vi "FVT (New Counter).vi"() -> ()   [LabVIEW 2024]
uses:
  Agilent 532XX Series/Public/Configure/Measurement/Configure Measurement (Frequency).vi
  <vilib>/Utility/file.llb/Write Delimited Spreadsheet (string).vi
  Agilent 532XX Series/Agilent 532XX Series.lvlib
panel:
  out "FrequencyCounter":refnum<visa-resource-name>
  in  "CompRun":bool
  out "Channel(s) (out)":u16(ring) items=["1+2", "1", "2", "3"]
  in  "Single Func Test":bool=TRUE
  in  "Position":i32 min=0 max=64 step=32
  in  "Number of Cycles":i32
  in  "Warmup Data":string[](array[string])
  out "Nominal Frequency":string="XXXXX-XXX"
  in  "Warmup":bool=TRUE
  out "Soak Time":u16(ring) items=["10", "5", "15", "30", "60", "90", "120"]
  out "Starting Time":string
  in  "Slew Time":dbl=2.0 format="%#_13g"
  out "Time Left (Estimate)":string
  out "Time":dbl
  out "PDF Path":string
  out "Time Start":timestamp
  in  "Halt Run":bool=TRUE
  out "Gatetime":string
  out "Delay Time":dbl
  out "Work Order":string
  out "Unit_Number":string
  out "System":string
  out "Path":string
  out "Frequency Address":i16=8
  out "HP Switcher Address":i32=3
  out "Oven Address":i32
  out "Temperature Array":dbl[](array[numeric])
  out "Temp Type":i32 min=1 max=15 step=1
  in  "Serial Numbers":string[](array[string])
  out "All Data":string[][][](array[string])
  in  "System Status":string
  out "Chamber":cluster{"GPIB #":u8, "Address":u8}={"GPIB #"=0, "Address"=28}
  in  "Exit":bool=TRUE
  out "Functional Test Data":string
  in  "Number of Units":i32 min=0 max=64 step=32
  in  "Functional Test":bool=TRUE
  in  "Start run":bool=TRUE
  # "FVT Test Chamber 3"
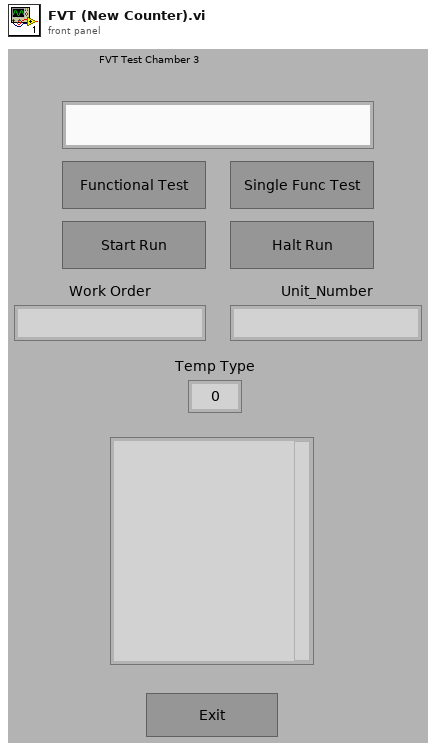
[diagram p1: front panel]
types:
  T1 = cluster{"GPIB Bus":i32, "HP Switcher Address":i32}
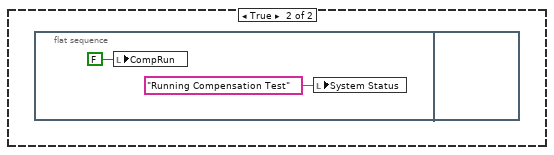
[diagram p2: hidden frame]
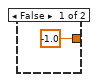
[diagram p4: hidden frame]
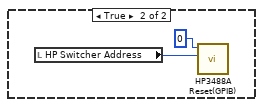
[diagram p5: hidden frame]
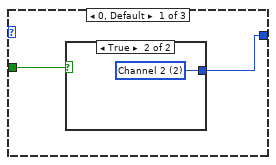
[diagram p6: hidden frame]
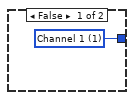
[diagram p7: hidden frame]
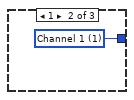
[diagram p8: hidden frame]
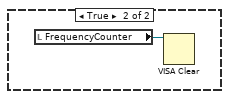
[diagram p9: hidden frame]
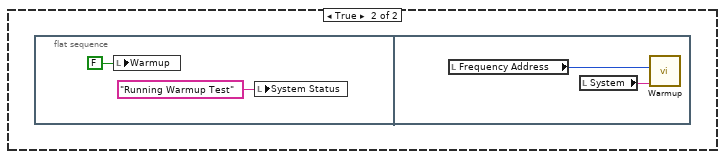
[diagram p10: hidden frame]
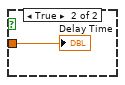
[diagram p12: hidden frame]
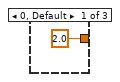
[diagram p13: hidden frame]
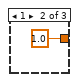
[diagram p14: hidden frame]
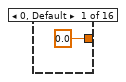
[diagram p16: hidden frame]
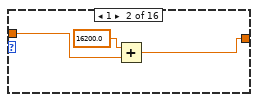
[diagram p17: hidden frame]
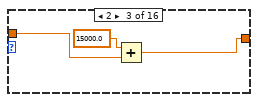
[diagram p18: hidden frame]
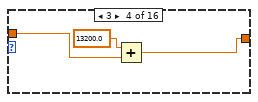
[diagram p19: hidden frame]
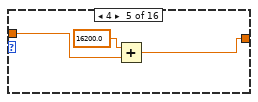
[diagram p20: hidden frame]
diagram:
  w2 = FALSE ("Exit")
  n1 = while {
    tunnel: [w16] -> w3
    stop <- w16 stop-if-true
    n2 = local read "CompRun"() -> (w11:bool)
    n3 = local write "Halt Run"(FALSE ("Halt Run")) -> ()
    n4 = local read "Start run"() -> (w18:bool)
    n5 = local read "Warmup"() -> (w13:bool)
    n6 = local read "Single Func Test"() -> (w12:bool)
    n7 = local read "Functional Test"() -> (w19:bool)
    n8 = local write "Time Left (Estimate)"("00:00:00" ("Time Left (Estimate)")) -> ()
    n9 = case shown="False" w11 {
      frame False {
      }
      frame True {
        n10 = flat-sequence {
          frame #0 {
            n11 = local write "CompRun"(FALSE ("CompRun")) -> ()
            n12 = local write "System Status"("Running Compensation Test" ("System Status")) -> ()
          }
          frame #1 {
          }
        }
      }
    }
    n13 = local write "System Status"("System Idle" ("System Status")) -> ()
    n14 = case shown="False" w13 {
      frame False {
      }
      frame True {
        n15 = flat-sequence {
          frame #0 {
            n16 = local write "Warmup"(FALSE ("Functional Test")) -> ()
            n17 = local write "System Status"("Running Warmup Test" ("System Status")) -> ()
          }
          frame #1 {
            n18 = local read "Frequency Address"() -> (w101:i16)
            n19 = local read "System"() -> (w102:string)
            n20 = call "Warmup.vi"("System"=w102, "Frequency Address"=w101) -> ()  [unwired: 10 in]
          }
        }
      }
    }
    n21 = case shown="True" w18 {
      frame False {
      }
      frame True {
        n22 = flat-sequence {
          frame #0 {
            n23 = Get Date/Time In Seconds() -> (seconds since 1Jan1904=w105:timestamp)
            n24 = Wait (ms)(milliseconds to wait=u32 5000) -> ()  [unwired: 1 out]
            n25 = Format Date/Time String(time format string (%c)="%c", seconds (now)=w105) -> (date/time string=→"Starting Time":string)  [unwired: 1 in]
            n26 = local write "System Status"("FVT running" ("System Status")) -> ()
          }
          frame #1 {
            n27 = flat-sequence {
              frame #0 {
                n28 = local read "HP Switcher Address"() -> (w109:i32)
                n29 = DevClear(3:w109, 4:0 ("GPIB Bus")) -> ()  [unwired: 1 in, 2 out]
              }
              frame #1 {
                n30 = local read "Oven Address"() -> (w111:i32)
                n31 = DevClear(3:w111, 4:0 ("GPIB Bus")) -> ()  [unwired: 1 in, 2 out]
              }
              frame #2 {
                n32 = local read "Frequency Address"() -> (w113:i16)
                n33 = DevClear(3:w113, 4:0 ("GPIB Bus")) -> ()  [unwired: 1 in, 2 out]
              }
            }
            n34 = local write "Start run"(FALSE ("Functional Test")) -> ()
          }
          frame #2 {
            n35 = call "Display Message to User"() -> ("Yes"=w125:bool)  [unwired: 10 in, 1 out]
            n36 = call "Prompt User for Input"("Enable"=w125) -> ("Seconds"=w123:dbl, "Minutes"=w119:dbl, "Hours"=w118:dbl)  [unwired: 14 in, 2 out]
            n37 = Multiply(x=w119, y=60.0) -> (x*y=w121:dbl)
            n38 = Multiply(x=w118, y=3600.0) -> (x*y=w120:dbl)
            n39 = Add(x=w120, y=w121) -> (x+y=w122:dbl)
            n40 = Add(x=w122, y=w123) -> (x+y=w124:dbl)
            n41 = Multiply(x=w124, y=1000.0) -> (x*y=w126:dbl)
            n42 = case shown="False" w125 {
              tunnel: w126 -> [_ w128]
              frame False {
                n43 = local write "Delay Time"(600000.0 ("Delay Time")) -> ()
              }
              frame True {
                "Delay Time" <- w128
              }
            }
          }
          frame #3 {
            n44 = call "Display Message to User"() -> ()  [unwired: 10 in, 2 out]
          }
          frame #4 {
            n45 = call "Parameter Setup.vi"() -> ("Serial Numbers"=w138:string[], "Slewtime (out)"=w132:u16, "Gatetime(out)"=w133:string, "Number of Units(out)"=w137:i32, "Soak Time(out)"=w130:u16, "Channel(s) (out)"=w129:u16, "Temp Type(out)"=w136:i32, "Unit_Number(out)"=w134:string, "Work Order(out)"=w135:string)  [unwired: 3 in]
            n46 = local write "Work Order"(w135) -> ()
            n47 = local write "Channel(s) (out)"(w129) -> ()
            n48 = local write "Number of Units"(w137) -> ()
            n49 = local write "Gatetime"(w133) -> ()
            n50 = case shown="2" w132 {
              tunnel: [2.0 ("Slew Time") 1.0 ("Slew Time") 0.5 ("Slew Time")] -> w131
              frame 0, Default {
              }
              frame 1 {
              }
              frame 2 {
              }
            }
            n51 = local write "Serial Numbers"(w138) -> ()
            n52 = local write "Soak Time"(w130) -> ()
            n53 = local write "Temp Type"(w136) -> ()
            n54 = local write "Unit_Number"(w134) -> ()
            n55 = local write "Slew Time"(w131) -> ()
          }
          frame #5 {
            n56 = Wait (ms)(milliseconds to wait=u32 500) -> ()  [unwired: 1 out]
          }
          frame #6 {
            w143 = "-" ("string")
            n57 = Get Date/Time In Seconds() -> (seconds since 1Jan1904=w154:timestamp)
            n58 = Format Date/Time String(time format string (%c)="%x_%I-%M" ("string"), seconds (now)=w154) -> (date/time string=w155:string)  [unwired: 1 in]
            n59 = local read "Unit_Number"() -> (w158:string)
            n60 = local read "Work Order"() -> (w157:string)
            n61 = Search and Replace String(replace all?=TRUE ("replace all? (F)"), input string=w155, search string="/", replace string="-" ("replace string (\"\")")) -> (result string=w156:string)  [unwired: 4 in, 3 out]
            n62 = Concatenate Strings("\\\\Bti-dc1\\ATE-Archive\\NewDataArchive\\_FvT\\" ("string"), "FVT-" ("string"), w157, w143, w158, w143, w156) -> (w150:string)
            n63 = local write "Path"(w150) -> ()
            n64 = String To Path(string=w150) -> (path=w151:path)
            n65 = call <vilib>:"Check if File or Folder Exists.vi"("path"=w151) -> ("file or folder exists?"=w152:bool, "dup path"=w153:path)  [unwired: 8 in, 1 out]
            n66 = case shown="False" w152 {
              tunnel: w153 -> [w159 _]
              frame False {
                n67 = Create Folder(path (use dialog)=w159) -> ()  [unwired: 2 in, 3 out]
              }
              frame True {
              }
            }
          }
          frame #7 {
            n68 = Wait (ms)(milliseconds to wait=u32 1000) -> ()  [unwired: 1 out]
          }
          frame #8 {
            n69 = flat-sequence {
              tunnel: [w166] -> w162
              tunnel: [w225] -> w161
              tunnel: w162 -> [w215]
              tunnel: w161 -> [w233]
              frame #0 {
                n70 = Get Date/Time In Seconds() -> (seconds since 1Jan1904=w167:timestamp)
                n71 = local read "Delay Time"() -> (w165:dbl)
                n72 = local write "Time Start"(w167) -> ()
                n73 = Divide(x=w165, y=1000.0) -> (x/y=w163:dbl)
                n74 = local read "Temp Type"() -> (w166:i32)
                n75 = case shown="15" w166 {
                  tunnel: w163 -> [_ w172 w175 w177 w181 w184 w187 w190 w193 w196 w199 w202 w205 w208 w211 w214]
                  tunnel: [0.0 ("Delay Time") w171 w174 w178 w180 w183 w186 w189 w192 w194 w197 w200 w203 w206 w209 w212] -> w168
                  frame 0, Default {
                  }
                  frame 1 {
                    n76 = Add(x=16200.0 ("Delay Time"), y=w172) -> (x+y=w171:dbl)
                  }
                  frame 2 {
                    n77 = Add(x=15000.0 ("Delay Time"), y=w175) -> (x+y=w174:dbl)
                  }
                  frame 3 {
                    n78 = Add(x=13200.0 ("Delay Time"), y=w177) -> (x+y=w178:dbl)
                  }
                  frame 4 {
                    n79 = Add(x=16200.0 ("Delay Time"), y=w181) -> (x+y=w180:dbl)
                  }
                  frame 5 {
                    n80 = Add(x=15000.0 ("Delay Time"), y=w184) -> (x+y=w183:dbl)
                  }
                  frame 6 {
                    n81 = Add(x=13200.0 ("Delay Time"), y=w187) -> (x+y=w186:dbl)
                  }
                  frame 7 {
                    n82 = Add(x=8400.0, y=w190) -> (x+y=w189:dbl)
                  }
                  frame 8 {
                    n83 = Add(x=14400.0 ("Delay Time"), y=w193) -> (x+y=w192:dbl)
                  }
                  frame 9 {
                    n84 = Add(x=16200.0 ("Delay Time"), y=w196) -> (x+y=w194:dbl)
                  }
                  frame 10 {
                    n85 = Add(x=15000.0 ("Delay Time"), y=w199) -> (x+y=w197:dbl)
                  }
                  frame 11 {
                    n86 = Add(x=15000.0 ("Delay Time"), y=w202) -> (x+y=w200:dbl)
                  }
                  frame 12 {
                    n87 = Add(x=15000.0 ("Delay Time"), y=w205) -> (x+y=w203:dbl)
                  }
                  frame 13 {
                    n88 = Add(x=15000.0 ("Delay Time"), y=w208) -> (x+y=w206:dbl)
                  }
                  frame 14 {
                    n89 = Add(x=15000.0 ("Delay Time"), y=w211) -> (x+y=w209:dbl)
                  }
                  frame 15 {
                    n90 = Add(x=15000.0 ("Delay Time"), y=w214) -> (x+y=w212:dbl)
                  }
                }
                "Time" <- w168
              }
              frame #1 {
                n91 = Number To Decimal String(number=w215) -> (decimal integer string=w224:string)  [unwired: 1 in]
                n92 = Concatenate Strings("\\\\BTI-dc1\\ATE\\Temp Tables\\" ("search string/char (-)"), w224, ".txt" ("string")) -> (w221:string)
                n93 = String To Path(string=w221) -> (path=w220:path)
                n94 = Read from Text File(file (use dialog)=w220, count=-1) -> (text=w219:string)  [unwired: 2 in, 3 out]
                n95 = while {
                  tunnel: [w230] -> w217 mode=indexing
                  shift-right: [w229] -> _
                  shift-left: w219 -> [w228]
                  stop <- w231 stop-if-true
                  n96 = Match Pattern(string=w228, regular expression="," ("search string/char (-)")) -> (before substring=w230:string, after substring=w229:string, offset past match=w226:i32)  [unwired: 1 in, 1 out]
                  n97 = Equal?(x=w226, y=-1) -> (x = y?=w231:bool)
                }
                n98 = Fract/Exp String To Number(string=w217) -> (number=w216:dbl[])  [unwired: 3 in, 1 out]
                "Temperature Array" <- w216
                n99 = Array Size(array=w216) -> (size(s)=w225:i32)
              }
              frame #2 {
                n100 = for {
                  N: w233 -> [_]
                  i -> [w235]
                  stop <- w234 stop-if-true
                  n101 = flat-sequence {
                    tunnel: w235 -> [w237]
                    tunnel: w235 -> [w490]
                    tunnel: w235 -> [w491]
                    frame #0 {
                      n102 = local read "Temperature Array"() -> (w243:dbl[])
                      n103 = Equal?(x=w237, y=0) -> (x = y?=w236:bool)
                      n104 = Index Array(array=w243, index=w237) -> (element=w239:dbl)
                      n105 = Number To Fractional String(number=w239) -> (F-format string=w241:string)  [unwired: 3 in]
                      n106 = case shown="False" w236 {
                        tunnel: w239 -> [w246 w338]
                        frame True {
                          n107 = flat-sequence {
                            tunnel: w246 -> [w260]
                            tunnel: [w260] -> w251
                            tunnel: [w278] -> w250
                            tunnel: [w277] -> w249
                            tunnel: w251 -> [w278]
                            tunnel: w250 -> [w284]
                            tunnel: [w284] -> w248
                            tunnel: w249 -> [w283]
                            tunnel: [w280] -> w244
                            tunnel: [w291] -> w247
                            tunnel: w248 -> [w291]
                            tunnel: [w290] -> w245
                            tunnel: w244 -> [w290]
                            tunnel: w247 -> [w294]
                            tunnel: w245 -> [w293]
                            frame #0 {
                              n108 = local read "Time Start"() -> (w258:timestamp)
                              n109 = Get Date/Time In Seconds() -> (seconds since 1Jan1904=w259:timestamp)
                              n110 = Subtract(x=w259, y=w258) -> (x-y=w256:dbl)
                              n111 = local read "Time"() -> (w255:dbl)
                              n112 = Subtract(x=w255, y=w256) -> (x-y=w253:dbl)
                              n113 = Less?(x=w253, y=0.0) -> (x < y?=w252:bool)
                              n114 = case shown="False" w252 {
                                tunnel: [w272 "00:00:00" ("time string")] -> w254
                                tunnel: w253 -> [w275 _]
                                frame False {
                                w273 = ":" ("string")
                                n115 = Quotient & Remainder(x=w275, y=3600.0) -> (x-y*floor(x/y)=w269:dbl, floor(x/y)=w271:dbl)
                                n116 = Quotient & Remainder(x=w269, y=60.0) -> (x-y*floor(x/y)=w265:dbl, floor(x/y)=w267:dbl)
                                n117 = Number To Fractional String(number=w265, precision (6)=i16 0) -> (F-format string=w264:string)  [unwired: 2 in]
                                n118 = Number To Fractional String(number=w267, precision (6)=i16 0) -> (F-format string=w266:string)  [unwired: 2 in]
                                n119 = Number To Fractional String(number=w271, precision (6)=i16 0) -> (F-format string=w270:string)  [unwired: 2 in]
                                n120 = Concatenate Strings(w270, w273, w266, w273, w264) -> (w272:string)
                                }
                                frame True {
                                }
                              }
                              n121 = local write "Time Left (Estimate)"(w254) -> ()
                            }
                            frame #1 {
                              n122 = Number To Decimal String(number=w278) -> (decimal integer string=w277:string)  [unwired: 1 in]
                            }
                            frame #2 {
                              n123 = local read "Oven Address"() -> (w279:i32)
                              n124 = Bundle(0, "Oven Address"=w279) -> (w281:cluster{i32, "Oven Address":i32})  [unwired: 1 in]
                              n125 = while {
                                tunnel: w283 -> [w289]
                                tunnel: w281 -> [w286]
                                tunnel: [w286] -> w280
                                stop <- w287 continue-if-true
                                n126 = call "Set Temperature and Rise Time2023.vi"("Slew Time String"="0", "Temperature String"=w289, "Device"=w286) -> ("error out"=w288:errorcluster)  [unwired: 3 in]
                                n127 = Unbundle By Name(w288) -> ("status"=w287:bool)
                              }
                            }
                            frame #3 {
                              n128 = Wait (ms)(milliseconds to wait=u32 1000) -> ()  [unwired: 1 out]
                            }
                            frame #4 {
                              n129 = while {
                                tunnel: w294 -> [w298]
                                tunnel: w293 -> [w295]
                                stop <- w296 stop-if-true
                                n130 = flat-sequence {
                                tunnel: w298 -> [w308]
                                tunnel: [w300] -> w297
                                tunnel: w295 -> [w299]
                                tunnel: w297 -> [w337]
                                tunnel: [w336] -> w296
                                frame #0 {
                                n131 = call "Read Saunders Temperature2023.vi"("Device"=w299) -> ("error out 2"=w301:errorcluster, "Temperature"=w303:dbl)  [unwired: 3 in]
                                n132 = Add(x=0.5, y=w308) -> (x+y=w304:dbl)
                                n133 = Subtract(x=w308, y=0.5) -> (x-y=w306:dbl)
                                n134 = Unbundle By Name(w301) -> ("status"=w302:bool)
                                n135 = In Range and Coerce(upper limit=w304, x=w303, lower limit=w306) -> (In Range?=w300:bool)  [unwired: 1 out]
                                n136 = case shown="False" w302 {
                                frame False {
                                }
                                frame True {
                                n137 = local read "Oven Address"() -> (w309:i32)
                                n138 = DevClear(3:w309, 4:0 ("GPIB Bus")) -> ()  [unwired: 1 in, 2 out]
                                }
                                }
                                }
                                frame #1 {
                                n139 = local read "Time Start"() -> (w317:timestamp)
                                n140 = Get Date/Time In Seconds() -> (seconds since 1Jan1904=w318:timestamp)
                                n141 = Subtract(x=w318, y=w317) -> (x-y=w315:dbl)
                                n142 = local read "Time"() -> (w316:dbl)
                                n143 = Subtract(x=w316, y=w315) -> (x-y=w312:dbl)
                                n144 = Less?(x=w312, y=0.0) -> (x < y?=w313:bool)
                                n145 = case shown="False" w313 {
                                tunnel: [w330 "00:00:00" ("time string")] -> w311
                                tunnel: w312 -> [w333 _]
                                frame False {
                                w331 = ":" ("string")
                                n146 = Quotient & Remainder(x=w333, y=3600.0) -> (x-y*floor(x/y)=w327:dbl, floor(x/y)=w329:dbl)
                                n147 = Quotient & Remainder(x=w327, y=60.0) -> (x-y*floor(x/y)=w323:dbl, floor(x/y)=w325:dbl)
                                n148 = Number To Fractional String(number=w323, precision (6)=i16 0) -> (F-format string=w322:string)  [unwired: 2 in]
                                n149 = Number To Fractional String(number=w325, precision (6)=i16 0) -> (F-format string=w324:string)  [unwired: 2 in]
                                n150 = Number To Fractional String(number=w329, precision (6)=i16 0) -> (F-format string=w328:string)  [unwired: 2 in]
                                n151 = Concatenate Strings(w328, w331, w324, w331, w322) -> (w330:string)
                                }
                                frame True {
                                }
                                }
                                n152 = local write "Time Left (Estimate)"(w311) -> ()
                                }
                                frame #2 {
                                n153 = local read "Halt Run"() -> (w335:bool)
                                n154 = Or(x=w335, y=w337) -> (x .or. y?=w336:bool)
                                }
                                }
                              }
                            }
                          }
                        }
                        frame False {
                          n155 = flat-sequence {
                            tunnel: w338 -> [w363]
                            tunnel: [w363] -> w354
                            tunnel: [w387] -> w353
                            tunnel: [w386] -> w352
                            tunnel: [w381] -> w351
                            tunnel: [w385] -> w350
                            tunnel: w354 -> [w387]
                            tunnel: w353 -> [w407]
                            tunnel: [w407] -> w349
                            tunnel: [w408] -> w348
                            tunnel: w352 -> [w410]
                            tunnel: [w410] -> w347
                            tunnel: w351 -> [w409]
                            tunnel: w350 -> [w406]
                            tunnel: [w431] -> w346
                            tunnel: w349 -> [w430]
                            tunnel: w348 -> [w429]
                            tunnel: w347 -> [w431]
                            tunnel: [w430] -> w345
                            tunnel: [w429] -> w344
                            tunnel: [w428] -> w343
                            tunnel: w346 -> [w432]
                            tunnel: [w432] -> w342
                            tunnel: w345 -> [w435]
                            tunnel: [w435] -> w341
                            tunnel: w344 -> [w434]
                            tunnel: w343 -> [w433]
                            tunnel: [w442] -> w340
                            tunnel: w342 -> [w442]
                            tunnel: [w441] -> w339
                            tunnel: w341 -> [w441]
                            tunnel: w340 -> [w445]
                            tunnel: w339 -> [w444]
                            frame #0 {
                              n156 = local read "Time Start"() -> (w361:timestamp)
                              n157 = Get Date/Time In Seconds() -> (seconds since 1Jan1904=w362:timestamp)
                              n158 = Subtract(x=w362, y=w361) -> (x-y=w358:dbl)
                              n159 = local read "Time"() -> (w359:dbl)
                              n160 = Subtract(x=w359, y=w358) -> (x-y=w355:dbl)
                              n161 = Less?(x=w355, y=0.0) -> (x < y?=w356:bool)
                              n162 = case shown="False" w356 {
                                tunnel: [w375 "00:00:00" ("time string")] -> w357
                                tunnel: w355 -> [w378 _]
                                frame False {
                                w376 = ":" ("string")
                                n163 = Quotient & Remainder(x=w378, y=3600.0) -> (x-y*floor(x/y)=w372:dbl, floor(x/y)=w374:dbl)
                                n164 = Quotient & Remainder(x=w372, y=60.0) -> (x-y*floor(x/y)=w368:dbl, floor(x/y)=w370:dbl)
                                n165 = Number To Fractional String(number=w368, precision (6)=i16 0) -> (F-format string=w367:string)  [unwired: 2 in]
                                n166 = Number To Fractional String(number=w370, precision (6)=i16 0) -> (F-format string=w369:string)  [unwired: 2 in]
                                n167 = Number To Fractional String(number=w374, precision (6)=i16 0) -> (F-format string=w373:string)  [unwired: 2 in]
                                n168 = Concatenate Strings(w373, w376, w369, w376, w367) -> (w375:string)
                                }
                                frame True {
                                }
                              }
                              n169 = local write "Time Left (Estimate)"(w357) -> ()
                            }
                            frame #1 {
                              n170 = local read "Oven Address"() -> (w380:i32)
                              n171 = Bundle(0, "Oven Address"=w380) -> (w386:cluster{i32, "Oven Address":i32})  [unwired: 1 in]
                              n172 = call "Read Saunders Temperature2023.vi"("Device"=w386) -> ("error out 2"=w383:errorcluster, "Temperature"=w382:dbl)  [unwired: 3 in]
                              n173 = Unbundle By Name(w383) -> ("status"=w384:bool)
                              n174 = case shown="False" w384 {
                                tunnel: w382 -> [w399 w404]
                                tunnel: [w399 w401] -> w381
                                frame False {
                                }
                                frame True {
                                n175 = In Range and Coerce(upper limit=100.0, x=w404, lower limit=-50.0) -> (coerced(x)=w401:dbl)  [unwired: 1 out]
                                n176 = local read "Oven Address"() -> (w400:i32)
                                n177 = DevClear(3:w400, 4:0 ("GPIB Bus")) -> ()  [unwired: 1 in, 2 out]
                                }
                              }
                              n178 = Greater?(x=w387, y=0) -> (0:w395:bool)
                              n179 = Less?(x=w387, y=0.0) -> (x < y?=w392:bool)
                              n180 = Less?(x=w381, y=0.0) -> (x < y?=w394:bool)
                              n181 = Greater?(x=w381, y=0.0) -> (0:w393:bool)
                              n182 = And(x=w395, y=w394) -> (x .and. y?=w391:bool)
                              n183 = And(x=w393, y=w392) -> (x .and. y?=w388:bool)
                              n184 = Or(x=w391, y=w388) -> (x .or. y?=w385:bool)
                            }
                            frame #2 {
                              n185 = case shown="True" w406 {
                                tunnel: w409 -> [w416 w424]
                                tunnel: w407 -> [w417 w425]
                                tunnel: [w413 w421] -> w408
                                frame False {
                                n186 = Subtract(x=w417, y=w416) -> (x-y=w415:dbl)
                                n187 = local read "Slew Time"() -> (w411:dbl)
                                n188 = Absolute Value(x=w415) -> (abs(x)=w412:dbl)
                                n189 = Quotient & Remainder(x=w412, y=w411) -> (floor(x/y)=w414:dbl)  [unwired: 1 out]
                                n190 = Number To Decimal String(number=w414) -> (decimal integer string=w413:string)  [unwired: 1 in]
                                }
                                frame True {
                                n191 = Absolute Value(x=w425) -> (abs(x)=w422:dbl)
                                n192 = Absolute Value(x=w424) -> (abs(x)=w423:dbl)
                                n193 = local read "Slew Time"() -> (w418:dbl)
                                n194 = Add(x=w422, y=w423) -> (x+y=w419:dbl)
                                n195 = Quotient & Remainder(x=w419, y=w418) -> (floor(x/y)=w420:dbl)  [unwired: 1 out]
                                n196 = Number To Decimal String(number=w420) -> (decimal integer string=w421:string)  [unwired: 1 in]
                                }
                              }
                            }
                            frame #3 {
                              n197 = local read "Oven Address"() -> (w426:i32)
                              n198 = Number To Decimal String(number=w430) -> (decimal integer string=w428:string)  [unwired: 1 in]
                              n199 = DevClear(3:w426, 4:0 ("GPIB Bus")) -> ()  [unwired: 1 in, 2 out]
                            }
                            frame #4 {
                              n200 = while {
                                tunnel: w434 -> [w440]
                                tunnel: w433 -> [w439]
                                tunnel: w432 -> [w438]
                                stop <- w436 continue-if-true
                                n201 = call "Set Temperature and Rise Time2023.vi"("Slew Time String"=w440, "Temperature String"=w439, "Device"=w438) -> ("error out"=w437:errorcluster)  [unwired: 3 in]
                                n202 = Unbundle By Name(w437) -> ("status"=w436:bool)
                              }
                            }
                            frame #5 {
                              n203 = Wait (ms)(milliseconds to wait=u32 1000) -> ()  [unwired: 1 out]
                            }
                            frame #6 {
                              n204 = while {
                                tunnel: w445 -> [w448]
                                tunnel: w444 -> [w449]
                                stop <- w446 stop-if-true
                                n205 = flat-sequence {
                                tunnel: w449 -> [w459]
                                tunnel: w448 -> [w454]
                                tunnel: [w450] -> w447
                                tunnel: w447 -> [w488]
                                tunnel: [w487] -> w446
                                frame #0 {
                                n206 = call "Read Saunders Temperature2023.vi"("Device"=w454) -> ("error out 2"=w451:errorcluster, "Temperature"=w453:dbl)  [unwired: 3 in]
                                n207 = Add(x=0.5, y=w459) -> (x+y=w455:dbl)
                                n208 = Subtract(x=w459, y=0.5) -> (x-y=w457:dbl)
                                n209 = Unbundle By Name(w451) -> ("status"=w452:bool)
                                n210 = In Range and Coerce(upper limit=w455, x=w453, lower limit=w457) -> (In Range?=w450:bool)  [unwired: 1 out]
                                n211 = case shown="False" w452 {
                                frame False {
                                }
                                frame True {
                                n212 = local read "Oven Address"() -> (w460:i32)
                                n213 = DevClear(3:w460, 4:0 ("GPIB Bus")) -> ()  [unwired: 1 in, 2 out]
                                }
                                }
                                }
                                frame #1 {
                                n214 = local read "Time Start"() -> (w468:timestamp)
                                n215 = Get Date/Time In Seconds() -> (seconds since 1Jan1904=w469:timestamp)
                                n216 = Subtract(x=w469, y=w468) -> (x-y=w465:dbl)
                                n217 = local read "Time"() -> (w466:dbl)
                                n218 = Subtract(x=w466, y=w465) -> (x-y=w462:dbl)
                                n219 = Less?(x=w462, y=0.0) -> (x < y?=w463:bool)
                                n220 = case shown="False" w463 {
                                tunnel: [w481 "00:00:00" ("time string")] -> w464
                                tunnel: w462 -> [w484 _]
                                frame False {
                                w482 = ":" ("string")
                                n221 = Quotient & Remainder(x=w484, y=3600.0) -> (x-y*floor(x/y)=w478:dbl, floor(x/y)=w480:dbl)
                                n222 = Quotient & Remainder(x=w478, y=60.0) -> (x-y*floor(x/y)=w474:dbl, floor(x/y)=w476:dbl)
                                n223 = Number To Fractional String(number=w474, precision (6)=i16 0) -> (F-format string=w473:string)  [unwired: 2 in]
                                n224 = Number To Fractional String(number=w476, precision (6)=i16 0) -> (F-format string=w475:string)  [unwired: 2 in]
                                n225 = Number To Fractional String(number=w480, precision (6)=i16 0) -> (F-format string=w479:string)  [unwired: 2 in]
                                n226 = Concatenate Strings(w479, w482, w475, w482, w473) -> (w481:string)
                                }
                                frame True {
                                }
                                }
                                n227 = local write "Time Left (Estimate)"(w464) -> ()
                                }
                                frame #2 {
                                n228 = local read "Halt Run"() -> (w486:bool)
                                n229 = Or(x=w486, y=w488) -> (x .or. y?=w487:bool)
                                }
                                }
                              }
                            }
                          }
                        }
                      }
                      n230 = Concatenate Strings("Setting Temperature to " ("System Status"), w241) -> (w240:string)
                      n231 = local write "System Status"(w240) -> ()
                    }
                    frame #1 {
                      n232 = local read "Halt Run"() -> (w489:bool)
                      n233 = case shown="False" w489 {
                        tunnel: w491 -> [w493 _]
                        tunnel: w490 -> [w492 _]
                        frame False {
                          n234 = flat-sequence {
                            tunnel: w493 -> [w495]
                            tunnel: w492 -> [w509]
                            frame #0 {
                              n235 = Equal?(x=w495, y=0) -> (x = y?=w494:bool)
                              n236 = case shown="True" w494 {
                                frame False {
                                }
                                frame True {
                                n237 = local read "Delay Time"() -> (w497:dbl)
                                n238 = Wait (ms)(milliseconds to wait=w497) -> ()  [unwired: 1 out]
                                }
                              }
                            }
                            frame #1 {
                              n239 = local read "Soak Time"() -> (w500:u16)
                              n240 = local read "HP Switcher Address"() -> (w499:i32)
                              n241 = case shown="2" w500 {
                                frame 0, Default {
                                n242 = Wait (ms)(milliseconds to wait=u32 600000) -> ()  [unwired: 1 out]
                                }
                                frame 1 {
                                n243 = Wait (ms)(milliseconds to wait=u32 300000) -> ()  [unwired: 1 out]
                                }
                                frame 2 {
                                n244 = Wait (ms)(milliseconds to wait=u32 10) -> ()  [unwired: 1 out]
                                }
                                frame 3 {
                                n245 = Wait (ms)(milliseconds to wait=u32 900000) -> ()  [unwired: 1 out]
                                }
                                frame 4 {
                                n246 = Wait (ms)(milliseconds to wait=u32 1800000) -> ()  [unwired: 1 out]
                                }
                                frame 5 {
                                n247 = Wait (ms)(milliseconds to wait=u32 3600000) -> ()  [unwired: 1 out]
                                }
                                frame 6 {
                                n248 = Wait (ms)(milliseconds to wait=u32 5400000) -> ()  [unwired: 1 out]
                                }
                                frame 7 {
                                n249 = Wait (ms)(milliseconds to wait=u32 7200000) -> ()  [unwired: 1 out]
                                }
                              }
                              n250 = call "HP3488A Reset(GPIB).vi"("Address"=w499, "GPIB#"=0 ("GPIB Bus")) -> ()  [unwired: 3 in, 1 out]
                            }
                            frame #2 {
                              n251 = local read "Number of Units"() -> (w511:i32)
                              n252 = local read "Serial Numbers"() -> (w510:string[])
                              n253 = for {
                                N: w511 -> [_]
                                tunnel: w510 -> [w518] mode=indexing
                                tunnel: w509 -> [w522]
                                i -> [w527]
                                stop <- w517 stop-if-true
                                n254 = Increment(x=w527) -> (x+1=w519:i32)
                                n255 = flat-sequence {
                                tunnel: w519 -> [w532]
                                tunnel: [w532] -> w516
                                tunnel: [w541] -> w515
                                tunnel: w516 -> [w541]
                                tunnel: w515 -> [w559]
                                tunnel: [w559] -> w514
                                tunnel: [w566] -> w526
                                tunnel: [w565] -> w525
                                tunnel: w514 -> [w566]
                                tunnel: [w571] -> w524
                                tunnel: w526 -> [w570]
                                tunnel: w524 -> [w637]
                                tunnel: [w637] -> w523
                                tunnel: w522 -> [w636]
                                tunnel: [w630] -> w521
                                tunnel: [w629] -> w520
                                tunnel: w519 -> [w631]
                                tunnel: w518 -> [w628]
                                tunnel: w523 -> [w661]
                                tunnel: w525 -> [w680]
                                tunnel: w518 -> [w665]
                                tunnel: w521 -> [w663]
                                tunnel: w520 -> [w673]
                                tunnel: [w667] -> w512
                                tunnel: [w681] -> w513
                                tunnel: w512 -> [w681]
                                tunnel: w513 -> [w683]
                                frame #0 {
                                n256 = Wait (ms)(milliseconds to wait=u32 1000) -> ()  [unwired: 1 out]
                                n257 = Number To Decimal String(number=w532) -> (decimal integer string=w529:string)  [unwired: 1 in]
                                n258 = Concatenate Strings("Reading for Position " ("System Status"), w529) -> (w528:string)
                                n259 = local write "System Status"(w528) -> ()
                                }
                                frame #1 {
                                n260 = local read "Time Start"() -> (w536:timestamp)
                                n261 = Get Date/Time In Seconds() -> (seconds since 1Jan1904=w540:timestamp)
                                n262 = Subtract(x=w540, y=w536) -> (x-y=w535:dbl)
                                n263 = local read "Time"() -> (w534:dbl)
                                n264 = Subtract(x=w534, y=w535) -> (x-y=w539:dbl)
                                n265 = Less?(x=w539, y=0.0) -> (x < y?=w537:bool)
                                n266 = case shown="False" w537 {
                                tunnel: [w553 "00:00:00" ("time string")] -> w533
                                tunnel: w539 -> [w556 _]
                                frame False {
                                w554 = ":" ("string")
                                n267 = Quotient & Remainder(x=w556, y=3600.0) -> (x-y*floor(x/y)=w550:dbl, floor(x/y)=w552:dbl)
                                n268 = Quotient & Remainder(x=w550, y=60.0) -> (x-y*floor(x/y)=w546:dbl, floor(x/y)=w548:dbl)
                                n269 = Number To Fractional String(number=w546, precision (6)=i16 0) -> (F-format string=w545:string)  [unwired: 2 in]
                                n270 = Number To Fractional String(number=w548, precision (6)=i16 0) -> (F-format string=w547:string)  [unwired: 2 in]
                                n271 = Number To Fractional String(number=w552, precision (6)=i16 0) -> (F-format string=w551:string)  [unwired: 2 in]
                                n272 = Concatenate Strings(w551, w554, w547, w554, w545) -> (w553:string)
                                }
                                frame True {
                                }
                                }
                                n273 = local write "Time Left (Estimate)"(w533) -> ()
                                }
                                frame #2 {
                                n274 = Wait (ms)(milliseconds to wait=u32 1000) -> ()  [unwired: 1 out]
                                }
                                frame #3 {
                                n275 = local read "Oven Address"() -> (w560:i32)
                                n276 = Bundle(0, "Oven Address"=w560) -> (w562:cluster{i32, "Oven Address":i32})  [unwired: 1 in]
                                n277 = call "Read Saunders Temperature2023.vi"("Device"=w562) -> ("error out 2"=w563:errorcluster, "Temperature"=w565:dbl)  [unwired: 3 in]
                                n278 = Unbundle By Name(w563) -> ("status"=w564:bool)
                                n279 = case shown="False" w564 {
                                frame False {
                                }
                                frame True {
                                n280 = local read "Oven Address"() -> (w567:i32)
                                n281 = DevClear(3:w567, 4:0 ("GPIB Bus")) -> ()  [unwired: 1 in, 2 out]
                                }
                                }
                                }
                                frame #4 {
                                n282 = for {
                                N: 10 -> [_]
                                tunnel: [w579] -> w571
                                tunnel: w570 -> [w578]
                                stop <- w573 stop-if-true
                                n283 = flat-sequence {
                                tunnel: w578 -> [w583]
                                tunnel: [w583] -> w581
                                tunnel: [w582] -> w577
                                tunnel: w581 -> [w594]
                                tunnel: [w594] -> w580
                                tunnel: [w601] -> w575
                                tunnel: [w620] -> w579
                                tunnel: w580 -> [w617]
                                frame #0 {
                                n284 = local read "HP Switcher Address"() -> (w587:i32)
                                n285 = Bundle(0, "HP Switcher Address"=w587) -> (w585:cluster{i32, "HP Switcher Address":i32})  [unwired: 1 in]
                                n286 = call "Close HP3488A Switcher(GPIB).vi"("Device In"=w585, "reset"=FALSE, "Use Card# 5"=TRUE, "ID query"=FALSE, "error in (no error)"=errorcluster {"status"=FALSE, "code"=0, "source"=""}, "Position Number"=w583) -> ("error out"=w584:errorcluster)  [unwired: 2 in]
                                n287 = Unbundle By Name(w584) -> ("status"=w582:bool)
                                n288 = case shown="True" w582 {
                                frame False {
                                }
                                frame True {
                                n289 = local read "HP Switcher Address"() -> (w592:i32)
                                n290 = call "HP3488A Reset(GPIB).vi"("Address"=w592, "GPIB#"=0 ("GPIB Bus")) -> ()  [unwired: 3 in, 1 out]
                                }
                                }
                                }
                                frame #1 {
                                n291 = Wait (ms)(milliseconds to wait=u32 1000) -> ()  [unwired: 1 out]
                                }
                                frame #2 {
                                n292 = local read "Channel(s) (out)"() -> (w613:u16)
                                n293 = Greater?(x=w617, y=16) -> (0:w602:bool)
                                n294 = case shown="0, Default" w613 {
                                tunnel: w602 -> [w622 _ _]
                                tunnel: [w621 w625 w626] -> w596
                                frame 0, Default {
                                n295 = case shown="False" w622 {
                                tunnel: [w623 w624] -> w621
                                frame False {
                                w623 = 1 items=["Channel 1"=1, "Channel 2"=2] ("Channel (1: Channel 1)")
                                }
                                frame True {
                                w624 = 2 items=["Channel 1"=1, "Channel 2"=2] ("Channel (1: Channel 1)")
                                }
                                }
                                }
                                frame 1 {
                                w625 = 1 items=["Channel 1"=1, "Channel 2"=2] ("Channel (1: Channel 1)")
                                }
                                frame 2 {
                                w626 = 2 items=["Channel 1"=1, "Channel 2"=2] ("Channel (1: Channel 1)")
                                }
                                }
                                n296 = local read "FrequencyCounter"() -> (w605:refnum<visa-resource-name>)
                                n297 = local read "Gatetime"() -> (w619:string)
                                n298 = Fract/Exp String To Number(string=w619) -> (number=w603:dbl)  [unwired: 3 in, 1 out]
                                n299 = call "Initialize.vi"("VISA resource name"=w605) -> ("error out"=w610:errorcluster, "VISA resource name out"=w611:refnum<visa-resource-name>)  [unwired: 9 in]
                                n300 = call "Configure Frequency Gate.vi"("error in (no error)"=w610, "Time Resolution (0.1 s)"=w603, "VISA resource name"=w611) -> ("error out"=w597:errorcluster, "VISA resource name out"=w600:refnum<visa-resource-name>)  [unwired: 7 in]
                                n301 = call-poly "Configure Measurement.vi"("error in (no error)"=w597, "Channel (1:Channel 1)"=w596, "VISA resource name"=w600) -> ("error out"=w598:errorcluster, "VISA resource name out"=w599:refnum<visa-resource-name>)  [unwired: 2 in, 5 out]
                                n302 = call "Read Measurement (Single).vi"("error in (no error)"=w598, "VISA resource name"=w599) -> ("error out"=w608:errorcluster, "Measurement"=w607:dbl, "VISA resource name out"=w609:refnum<visa-resource-name>)  [unwired: 7 in]
                                n303 = call "Close.vi"("error in (no error)"=w608, "VISA resource name"=w609) -> ("error out"=w606:errorcluster)  [unwired: 9 in]
                                n304 = In Range and Coerce(upper limit=5000000000.0, x=w607, lower limit=0.0) -> (coerced(x)=w604:dbl)  [unwired: 1 out]
                                n305 = Unbundle By Name(w606) -> ("status"=w616:bool)
                                n306 = case shown="True" w616 {
                                frame False {
                                }
                                frame True {
                                n307 = local read "FrequencyCounter"() -> (w627:refnum<visa-resource-name>)
                                n308 = VISA Clear(VISA resource name=w627) -> ()  [unwired: 1 in, 2 out]
                                }
                                }
                                n309 = Not Equal?(x=w607, y=0.0) -> (x != y?=w601:bool)
                                n310 = Number To Fractional String(number=w604) -> (F-format string=w620:string)  [unwired: 3 in]
                                }
                                }
                                n311 = Not(x=w577) -> (.not. x?=w576:bool)
                                n312 = local read "Halt Run"() -> (w572:bool)
                                n313 = And(x=w575, y=w576) -> (x .and. y?=w574:bool)
                                n314 = Or(x=w574, y=w572) -> (x .or. y?=w573:bool)
                                }
                                }
                                frame #5 {
                                n315 = local read "Path"() -> (w635:string)
                                n316 = Concatenate Strings(w635, "\\" ("string"), w628, ".csv" ("string")) -> (w632:string)
                                n317 = String To Path(string=w632) -> (path=w629:path)
                                n318 = case shown="0" w636 {
                                tunnel: w629 -> [w653 _]
                                frame 0 {
                                n319 = Build Array("Unit_Number" ("string"), "Serial_Number" ("element"), "Date_Code" ("element"), "Work_Order" ("element"), "Test_System" ("element"), "Position" ("element"), "Fixture_SN" ("element"), "Run_FileName" ("element"), "Frequency" ("element"), "Temperature" ("element"), "Time_stamp" ("element"), "Run_ID" ("element")) -> (w652:string[])
                                n320 = call-poly <vilib>:"Write Delimited Spreadsheet.vi"("file path (dialog if empty)"=w653, "1D data"=w652, "append to file? (new file:F)"=FALSE, "delimiter (\\t)"="," ("delimiter (\\t)")) -> ()  [unwired: 10 in, 2 out]
                                }
                                frame 1, Default {
                                }
                                }
                                n321 = Number To Decimal String(number=w631) -> (decimal integer string=w630:string)  [unwired: 1 in]
                                }
                                frame #6 {
                                w656 = "','" ("element")
                                n322 = Get Date/Time In Seconds() -> (seconds since 1Jan1904=w679:timestamp)
                                n323 = local read "Temp Type"() -> (w669:i32)
                                n324 = local read "Slew Time"() -> (w668:dbl)
                                n325 = local read "Unit_Number"() -> (w662:string)
                                n326 = local read "Starting Time"() -> (w655:string)
                                n327 = local read "Work Order"() -> (w678:string)
                                n328 = Format Date/Time String(time format string (%c)="%c", seconds (now)=w679) -> (date/time string=w657:string)  [unwired: 1 in]
                                n329 = Number To Fractional String(number=w680) -> (F-format string=w660:string)  [unwired: 3 in]
                                n330 = Number To Decimal String(number=w669) -> (decimal integer string=w659:string)  [unwired: 1 in]
                                n331 = Number To Fractional String(number=w668) -> (F-format string=w658:string)  [unwired: 3 in]
                                n332 = local read "System"() -> (w664:string)
                                n333 = Concatenate Strings("INSERT INTO FVT\nVALUES('" ("element"), w665, w656, w662, w656, w664, w656, w663, w656, w662, w656, w661, w656, w660, w656, w659, w656, w658, w656, w657, w656, w655, "')" ("Unit_Number")) -> (w667:string)
                                n334 = Build Array(w662, w665, w665, w678, w664, w663, "" ("element"), "NONE" ("element"), w661, w660, w657, "1313" ("element")) -> (w670:string[])
                                n335 = call-poly <vilib>:"Write Delimited Spreadsheet.vi"("file path (dialog if empty)"=w673, "1D data"=w670, "append to file? (new file:F)"=TRUE, "delimiter (\\t)"="," ("delimiter (\\t)")) -> ()  [unwired: 10 in, 2 out]
                                }
                                frame #7 {
                                n336 = Wait (ms)(milliseconds to wait=u32 500) -> ()  [unwired: 1 out]
                                }
                                frame #8 {
                                n337 = call "Database Sending.vi"("Command"=w683) -> ()  [unwired: 11 in]
                                }
                                }
                                n338 = local read "Halt Run"() -> (w517:bool)
                              }
                            }
                          }
                        }
                        frame True {
                        }
                      }
                    }
                  }
                  n339 = local read "Halt Run"() -> (w234:bool)
                }
              }
            }
          }
          frame #9 {
            n340 = local read "Oven Address"() -> (w685:i32)
            n341 = Bundle(0, "Oven Address"=w685) -> (w684:cluster{i32, "Oven Address":i32})  [unwired: 1 in]
            n342 = call "Set Temperature and Rise Time2023.vi"("Temperature String"="O", "Device"=w684) -> ()  [unwired: 4 in, 1 out]
          }
          frame #10 {
            n343 = local read "Halt Run"() -> (w689:bool)
            n344 = Not(x=w689) -> (.not. x?=w688:bool)
            n345 = case shown="True" w688 {
              frame False {
              }
              frame True {
                n346 = local read "Number of Units"() -> (w690:i32)
                n347 = for {
                  N: w690 -> [_]
                  i -> [w692]
                  n348 = flat-sequence {
                    tunnel: w692 -> [w705]
                    tunnel: [w703] -> w691
                    tunnel: w691 -> [w719]
                    frame #0 {
                      n349 = Wait (ms)(milliseconds to wait=u32 1000) -> ()  [unwired: 1 out]
                      n350 = local write "System Status"("Converting Files to Winplot PDFs") -> ()
                    }
                    frame #1 {
                      w696 = "-" ("string")
                      n351 = Get Date/Time In Seconds() -> (seconds since 1Jan1904=w702:timestamp)
                      n352 = Format Date/Time String(time format string (%c)="%x_%I-%M" ("string"), seconds (now)=w702) -> (date/time string=w698:string)  [unwired: 1 in]
                      n353 = local read "Serial Numbers"() -> (w706:string[])
                      n354 = local read "Unit_Number"() -> (w714:string)
                      n355 = local read "Work Order"() -> (w715:string)
                      n356 = Search and Replace String(replace all?=TRUE ("replace all? (F)"), input string=w698, search string="/", replace string="-" ("replace string (\"\")")) -> (result string=w695:string)  [unwired: 4 in, 3 out]
                      n357 = Concatenate Strings("\\\\Bti-dc1\\ate\\Winplots\\" ("string"), "FVT-" ("string"), w715, w696, w714, w696, w695) -> (w708:string)
                      n358 = Index Array(array=w706, index=w705) -> (element=w703:string)
                      n359 = String To Path(string=w708) -> (path=w711:path)
                      n360 = call <vilib>:"Check if File or Folder Exists.vi"("path"=w711) -> ("file or folder exists?"=w712:bool, "dup path"=w713:path)  [unwired: 8 in, 1 out]
                      n361 = Concatenate Strings(w708, "\\" ("string"), w703) -> (w704:string)
                      n362 = case shown="False" w712 {
                        tunnel: w713 -> [w716 _]
                        frame False {
                          n363 = Create Folder(path (use dialog)=w716) -> ()  [unwired: 2 in, 3 out]
                        }
                        frame True {
                        }
                      }
                      n364 = local write "PDF Path"(w704) -> ()
                    }
                    frame #2 {
                      n365 = local read "Path"() -> (w721:string)
                      n366 = Concatenate Strings(w721, "\\" ("string"), w719, ".csv" ("string")) -> (w717:string)
                      n367 = local read "PDF Path"() -> (w730:string)
                      n368 = Open Python Session(python version="3.12" ("Python version")) -> (session out=w729:refnum<k35>, error out=w728:errorcluster)  [unwired: 2 in]
                      n369 = node(w729, path "C:/Users/presentation/Desktop/FVT FIXER/convert.py" ("module path"), "load_data" ("function name"), w728, string[] [], w717, w730) -> (w727:refnum<k35>, w726:errorcluster)  [unwired: 3 in, 2 out]
                      n370 = Close Python Session(session in=w727, error in=w726) -> ()  [unwired: 1 out]
                    }
                  }
                }
              }
            }
          }
          frame #11 {
            n371 = invoke on="Work Order" class="Str" method="Reinit To Default"() -> ()  [unwired: 3 in, 3 out]
            n372 = invoke on="Unit_Number" class="Str" method="Reinit To Default"() -> ()  [unwired: 3 in, 3 out]
            n373 = invoke on="Temp Type" class="DigNum (strict)" method="Reinit To Default"() -> ()  [unwired: 3 in, 3 out]
            n374 = local write "Halt Run"(FALSE ("Halt Run")) -> ()
          }
        }
      }
    }
    n375 = case shown="True" w12 {
      frame False {
      }
      frame True {
        n376 = flat-sequence {
          tunnel: [w27] -> w22
          tunnel: [w31] -> w23
          tunnel: w22 -> [w29]
          tunnel: w23 -> [w97]
          frame #0 {
            n377 = local write "Single Func Test"(FALSE ("Functional Test")) -> ()
            n378 = local write "System Status"("Running Single Functional Test" ("System Status")) -> ()
          }
          frame #1 {
            n379 = call "Parameter Setup( Single Functional).vi"() -> ("Run?"=w27:bool, "Position(out)"=w28:i32, "Channel(s) (out)"=w26:u16)  [unwired: 9 in]
            n380 = local write "Channel(s) (out)"(w26) -> ()
            n381 = local write "Position"(w28) -> ()
          }
          frame #2 {
            n382 = case shown="True" w29 {
              tunnel: [-1.0 ("upper limit") w33] -> w30
              frame False {
              }
              frame True {
                n383 = flat-sequence {
                  tunnel: [w43] -> w33
                  frame #0 {
                    n384 = Wait (ms)(milliseconds to wait=u32 500) -> ()  [unwired: 1 out]
                  }
                  frame #1 {
                    n385 = flat-sequence {
                      frame #0 {
                        n386 = local read "HP Switcher Address"() -> (w35:i32)
                        n387 = DevClear(3:w35, 4:0 ("GPIB Bus")) -> ()  [unwired: 1 in, 2 out]
                      }
                      frame #1 {
                        n388 = local read "Oven Address"() -> (w37:i32)
                        n389 = DevClear(3:w37, 4:0 ("GPIB Bus")) -> ()  [unwired: 1 in, 2 out]
                      }
                      frame #2 {
                        n390 = local read "Frequency Address"() -> (w39:i16)
                        n391 = DevClear(3:w39, 4:0 ("GPIB Bus")) -> ()  [unwired: 1 in, 2 out]
                      }
                    }
                  }
                  frame #2 {
                    n392 = Wait (ms)(milliseconds to wait=u32 100) -> ()  [unwired: 1 out]
                  }
                  frame #3 {
                    n393 = for {
                      N: 10 -> [_]
                      tunnel: [w50] -> w43
                      stop <- w44 stop-if-true
                      n394 = flat-sequence {
                        tunnel: [w53] -> w52
                        tunnel: [w54] -> w47
                        tunnel: [w65] -> w51
                        tunnel: w52 -> [w65]
                        tunnel: [w86] -> w50
                        tunnel: w51 -> [w85]
                        tunnel: [w83] -> w49
                        frame #0 {
                          n395 = local read "HP Switcher Address"() -> (w60:i32)
                          n396 = local read "Position"() -> (w53:i32)
                          n397 = Bundle("GPIB Bus"=0, "HP Switcher Address"=w60) -> (w61:T1)  [unwired: 1 in]
                          n398 = call "Close HP3488A Switcher(GPIB).vi"("Device In"=w61, "reset"=FALSE, "Use Card# 5"=TRUE, "ID query"=FALSE, "error in (no error)"=errorcluster {"status"=FALSE, "code"=0, "source"=""}, "Position Number"=w53) -> ("error out"=w62:errorcluster)  [unwired: 2 in]
                          n399 = Unbundle By Name(w62) -> ("status"=w54:bool)
                          n400 = case shown="False" w54 {
                            frame False {
                            }
                            frame True {
                              n401 = local read "HP Switcher Address"() -> (w63:i32)
                              n402 = call "HP3488A Reset(GPIB).vi"("Address"=w63, "GPIB#"=0 ("GPIB Bus")) -> ()  [unwired: 3 in, 1 out]
                            }
                          }
                        }
                        frame #1 {
                          n403 = Wait (ms)(milliseconds to wait=u32 500) -> ()  [unwired: 1 out]
                        }
                        frame #2 {
                          n404 = Greater?(x=w85, y=16) -> (0:w82:bool)
                          n405 = local read "Channel(s) (out)"() -> (w81:u16)
                          n406 = case shown="2" w81 {
                            tunnel: w82 -> [w91 _ _]
                            tunnel: [w90 w94 w95] -> w69
                            frame 0, Default {
                              n407 = case shown="True" w91 {
                                tunnel: [w92 w93] -> w90
                                frame False {
                                w92 = 1 items=["Channel 1"=1, "Channel 2"=2] ("Channel (1: Channel 1)")
                                }
                                frame True {
                                w93 = 2 items=["Channel 1"=1, "Channel 2"=2] ("Channel (1: Channel 1)")
                                }
                              }
                            }
                            frame 1 {
                              w94 = 1 items=["Channel 1"=1, "Channel 2"=2] ("Channel (1: Channel 1)")
                            }
                            frame 2 {
                              w95 = 2 items=["Channel 1"=1, "Channel 2"=2] ("Channel (1: Channel 1)")
                            }
                          }
                          n408 = local read "FrequencyCounter"() -> (w72:refnum<visa-resource-name>)
                          n409 = call "Initialize.vi"("VISA resource name"=w72) -> ("error out"=w78:errorcluster, "VISA resource name out"=w79:refnum<visa-resource-name>)  [unwired: 9 in]
                          n410 = call "Configure Frequency Gate.vi"("error in (no error)"=w78, "Time Resolution (0.1 s)"=0.1 ("Gate Time"), "VISA resource name"=w79) -> ("error out"=w70:errorcluster, "VISA resource name out"=w71:refnum<visa-resource-name>)  [unwired: 7 in]
                          n411 = call-poly "Configure Measurement.vi"("error in (no error)"=w70, "Channel (1:Channel 1)"=w69, "VISA resource name"=w71) -> ("error out"=w67:errorcluster, "VISA resource name out"=w68:refnum<visa-resource-name>)  [unwired: 2 in, 5 out]
                          n412 = call "Read Measurement (Single).vi"("error in (no error)"=w67, "VISA resource name"=w68) -> ("error out"=w76:errorcluster, "Measurement"=w74:dbl, "VISA resource name out"=w77:refnum<visa-resource-name>)  [unwired: 7 in]
                          n413 = call "Close.vi"("error in (no error)"=w76, "VISA resource name"=w77) -> ("error out"=w73:errorcluster)  [unwired: 9 in]
                          n414 = In Range and Coerce(upper limit=5000000000.0, x=w74, lower limit=0.0) -> (coerced(x)=w86:dbl)  [unwired: 1 out]
                          n415 = Unbundle By Name(w73) -> ("status"=w89:bool)
                          n416 = case shown="False" w89 {
                            frame False {
                            }
                            frame True {
                              n417 = local read "FrequencyCounter"() -> (w96:refnum<visa-resource-name>)
                              n418 = VISA Clear(VISA resource name=w96) -> ()  [unwired: 1 in, 2 out]
                            }
                          }
                          n419 = Not Equal?(x=w74, y=0.0) -> (x != y?=w83:bool)
                        }
                      }
                      n420 = Not(x=w47) -> (.not. x?=w48:bool)
                      n421 = local read "Halt Run"() -> (w46:bool)
                      n422 = And(x=w49, y=w48) -> (x .and. y?=w45:bool)
                      n423 = Or(x=w46, y=w45) -> (x .or. y?=w44:bool)
                    }
                  }
                }
              }
            }
            n424 = Number To Fractional String(number=w30) -> (F-format string=w31:string)  [unwired: 3 in]
          }
          frame #3 {
            n425 = local write "Functional Test Data"(w97) -> ()
            n426 = local write "Halt Run"(FALSE ("Halt Run")) -> ()
          }
        }
      }
    }
    n427 = case shown="True" w19 {
      frame False {
      }
      frame True {
        n428 = flat-sequence {
          tunnel: [w745] -> w732
          tunnel: w732 -> [w818]
          frame #0 {
            n429 = local write "Functional Test"(FALSE ("Functional Test")) -> ()
            n430 = local write "System Status"("Running Functional Test" ("System Status")) -> ()
          }
          frame #1 {
            n431 = call "Parameter Setup(Functional).vi"() -> ("Channel(s) (out)"=w735:u16, "Number of Units(out)"=w736:i32)  [unwired: 10 in]
            n432 = local write "Number of Units"(w736) -> ()
            n433 = local write "Channel(s) (out)"(w735) -> ()
          }
          frame #2 {
            n434 = Wait (ms)(milliseconds to wait=u32 500) -> ()  [unwired: 1 out]
          }
          frame #3 {
            n435 = flat-sequence {
              frame #0 {
                n436 = local read "HP Switcher Address"() -> (w738:i32)
                n437 = DevClear(3:w738, 4:0 ("GPIB Bus")) -> ()  [unwired: 1 in, 2 out]
              }
              frame #1 {
                n438 = local read "Oven Address"() -> (w740:i32)
                n439 = DevClear(3:w740, 4:0 ("GPIB Bus")) -> ()  [unwired: 1 in, 2 out]
              }
              frame #2 {
                n440 = local read "Frequency Address"() -> (w742:i16)
                n441 = DevClear(3:w742, 4:0 ("GPIB Bus")) -> ()  [unwired: 1 in, 2 out]
              }
            }
          }
          frame #4 {
            n442 = Wait (ms)(milliseconds to wait=u32 500) -> ()  [unwired: 1 out]
          }
          frame #5 {
            n443 = local read "Number of Units"() -> (w747:i32)
            n444 = for {
              N: w747 -> [_]
              shift-right: [w756] -> w745
              shift-left: "" -> [w755]
              i -> [w750]
              stop <- w748 stop-if-true
              n445 = Increment(x=w750) -> (x+1=w749:i32)
              n446 = flat-sequence {
                tunnel: w749 -> [w759]
                tunnel: [w759] -> w751
                tunnel: [w762] -> w757
                tunnel: w751 -> [w761]
                frame #0 {
                  n447 = Wait (ms)(milliseconds to wait=u32 100) -> ()  [unwired: 1 out]
                }
                frame #1 {
                  n448 = for {
                    N: 10 -> [_]
                    tunnel: w761 -> [w770]
                    tunnel: [w769] -> w762
                    stop <- w763 stop-if-true
                    n449 = flat-sequence {
                      tunnel: w770 -> [w774]
                      tunnel: [w774] -> w772
                      tunnel: [w773] -> w766
                      tunnel: [w785] -> w771
                      tunnel: w772 -> [w785]
                      tunnel: [w793] -> w769
                      tunnel: w771 -> [w808]
                      tunnel: [w792] -> w768
                      frame #0 {
                        n450 = local read "HP Switcher Address"() -> (w780:i32)
                        n451 = Bundle("GPIB Bus"=0, "HP Switcher Address"=w780) -> (w781:T1)  [unwired: 1 in]
                        n452 = call "Close HP3488A Switcher(GPIB).vi"("Device In"=w781, "reset"=FALSE, "Use Card# 5"=TRUE, "ID query"=FALSE, "error in (no error)"=errorcluster {"status"=FALSE, "code"=0, "source"=""}, "Position Number"=w774) -> ("error out"=w782:errorcluster)  [unwired: 2 in]
                        n453 = Unbundle By Name(w782) -> ("status"=w773:bool)
                        n454 = case shown="True" w773 {
                          frame False {
                          }
                          frame True {
                            n455 = local read "HP Switcher Address"() -> (w783:i32)
                            n456 = call "HP3488A Reset(GPIB).vi"("Address"=w783, "GPIB#"=0 ("GPIB Bus")) -> ()  [unwired: 3 in, 1 out]
                          }
                        }
                      }
                      frame #1 {
                        n457 = Wait (ms)(milliseconds to wait=u32 500) -> ()  [unwired: 1 out]
                      }
                      frame #2 {
                        n458 = Greater?(x=w808, y=16) -> (0:w794:bool)
                        n459 = local read "Channel(s) (out)"() -> (w804:u16)
                        n460 = case shown="1" w804 {
                          tunnel: w794 -> [w811 _ _]
                          tunnel: [w810 w814 w815] -> w787
                          frame 0, Default {
                            n461 = case shown="False" w811 {
                              tunnel: [w812 w813] -> w810
                              frame False {
                                w812 = 1 items=["Channel 1"=1, "Channel 2"=2] ("Channel (1: Channel 1)")
                              }
                              frame True {
                                w813 = 2 items=["Channel 1"=1, "Channel 2"=2] ("Channel (1: Channel 1)")
                              }
                            }
                          }
                          frame 1 {
                            w814 = 1 items=["Channel 1"=1, "Channel 2"=2] ("Channel (1: Channel 1)")
                          }
                          frame 2 {
                            w815 = 2 items=["Channel 1"=1, "Channel 2"=2] ("Channel (1: Channel 1)")
                          }
                        }
                        n462 = local read "FrequencyCounter"() -> (w795:refnum<visa-resource-name>)
                        n463 = call "Initialize.vi"("VISA resource name"=w795) -> ("error out"=w801:errorcluster, "VISA resource name out"=w802:refnum<visa-resource-name>)  [unwired: 9 in]
                        n464 = call "Configure Frequency Gate.vi"("error in (no error)"=w801, "Time Resolution (0.1 s)"=0.1 ("Gate Time"), "VISA resource name"=w802) -> ("error out"=w788:errorcluster, "VISA resource name out"=w791:refnum<visa-resource-name>)  [unwired: 7 in]
                        n465 = call-poly "Configure Measurement.vi"("error in (no error)"=w788, "Channel (1:Channel 1)"=w787, "VISA resource name"=w791) -> ("error out"=w789:errorcluster, "VISA resource name out"=w790:refnum<visa-resource-name>)  [unwired: 2 in, 5 out]
                        n466 = call "Read Measurement (Single).vi"("error in (no error)"=w789, "VISA resource name"=w790) -> ("error out"=w799:errorcluster, "Measurement"=w797:dbl, "VISA resource name out"=w800:refnum<visa-resource-name>)  [unwired: 7 in]
                        n467 = call "Close.vi"("error in (no error)"=w799, "VISA resource name"=w800) -> ("error out"=w796:errorcluster)  [unwired: 9 in]
                        n468 = In Range and Coerce(upper limit=5000000000.0, x=w797, lower limit=0.0) -> (coerced(x)=w793:dbl)  [unwired: 1 out]
                        n469 = Unbundle By Name(w796) -> ("status"=w807:bool)
                        n470 = case shown="True" w807 {
                          frame False {
                          }
                          frame True {
                            n471 = local read "FrequencyCounter"() -> (w816:refnum<visa-resource-name>)
                            n472 = VISA Clear(VISA resource name=w816) -> ()  [unwired: 1 in, 2 out]
                          }
                        }
                        n473 = Not Equal?(x=w797, y=0.0) -> (x != y?=w792:bool)
                      }
                    }
                    n474 = Not(x=w766) -> (.not. x?=w767:bool)
                    n475 = local read "Halt Run"() -> (w765:bool)
                    n476 = And(x=w768, y=w767) -> (x .and. y?=w764:bool)
                    n477 = Or(x=w765, y=w764) -> (x .or. y?=w763:bool)
                  }
                }
              }
              n478 = Number To Fractional String(number=w757) -> (F-format string=w754:string)  [unwired: 3 in]
              n479 = Concatenate Strings(w754, "\r\n") -> (w752:string)
              n480 = local read "Halt Run"() -> (w748:bool)
              n481 = Concatenate Strings(w755, w752) -> (w756:string)
            }
          }
          frame #6 {
            n482 = local write "Halt Run"(FALSE ("Halt Run")) -> ()
            "Functional Test Data" <- w818
          }
        }
      }
    }
    n483 = local read "Exit"() -> (w16:bool)
  }
  n484 = local write "Single Func Test"(w2) -> ()
  n485 = local write "Warmup"(w2) -> ()
  n486 = local write "Halt Run"(w2) -> ()
  n487 = local write "CompRun"(w2) -> ()
  n488 = local write "Start run"(w2) -> ()
  n489 = local write "Functional Test"(w2) -> ()
  n490 = local write "Exit"(w2) -> ()
  n491 = case shown="True" w3 {
    frame False {
    }
    frame True {
      n492 = invoke class="VI" method="FP.Close"() -> ()  [unwired: 3 in, 3 out]
    }
  }
  "Chamber" <- cluster{"GPIB #":u8, "Address":u8} {"GPIB #"=0, "Address"=6} ("Chamber")
  "All Data" <- string[][][] [] ("All Data")
  "Oven Address" <- 6 ("Oven Address")
  "HP Switcher Address" <- 3 ("Bliley Switcher Address")
  "Frequency Address" <- i16 8 ("Frequency Address")
  "System" <- "BTI-BILL3" ("System")
  "Gatetime" <- "1" ("Gatetime")
  "FrequencyCounter" <- refnum<visa-resource-name> "GPIB0::8::INSTR" ("FrequencyCounter")
